vi "S2C_PCIe7841_Proc_Globals.vi"() -> ()   [LabVIEW 2015]
panel:
  in  "ResourceName":string
  in  "FPGA_Ref":refnum<k20>
  out "Running?":bool
  out "7841-Errors":cluster{"Code":i32, "Source":string}[](array[cluster])=[{"Code"=6000, "Source"="A error occurred while attempting to send an event-level local command."}, {"Code"=6001, "Source"="A error occurred while attempting to clear the communications log."}]
  out "7841-Refs":string[][](array[string])
  in  "7841-VI":refnum<vi>
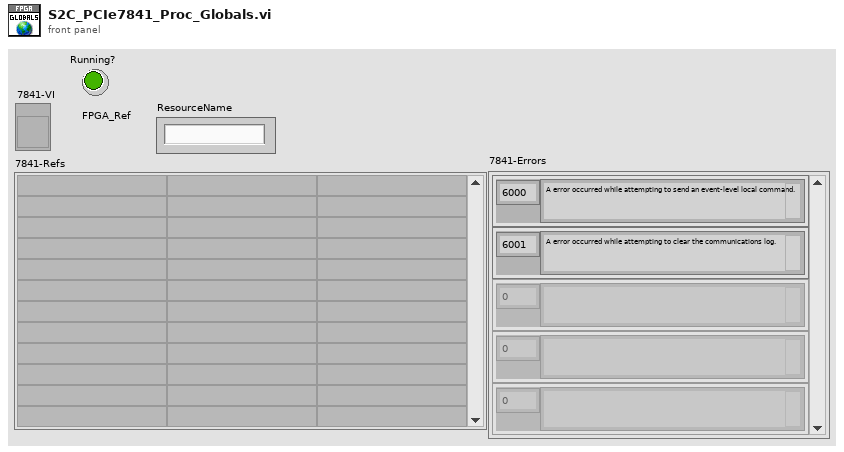
[diagram p1: front panel]
diagram:
